vi "Data entry form Post-Assembly.vi"(8 "error in (no error)":errorcluster, 10 "Stack names":T2, 11 "Database Entry in":refnum<class "Database Entry.lvclass">) -> (0 "error out":errorcluster, 2 "Post-Assembly Comments Out":T1, 3 "Database Entry out":refnum<class "Database Entry.lvclass">)   [LabVIEW 2021, in "Database Entry.lvclass"]
uses:
  Database Entry.lvclass
  Components/Stack/Stack.lvclass
panel:
  in  "Submit":bool
  in  "Post-Assembly Comments (If Any)":T3
  # "Note:\nEnsure 320P/320M in stack name to write to their respective tables.\nThis only updates existing \nstacks in postgres."
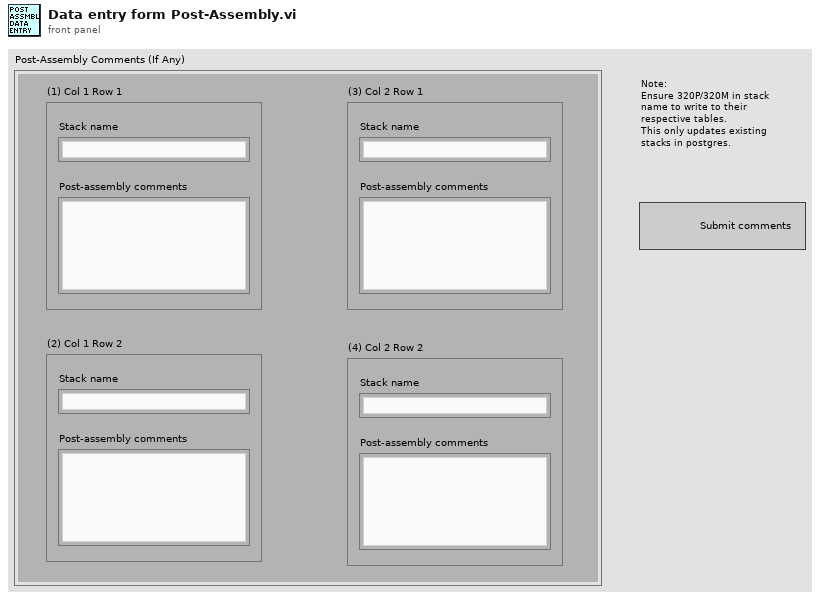
[diagram p1: front panel]
types:
  T1 = cluster{"(1) Tray 1 Pos 1":cluster{"Stack name":string, "Post-assembly comments":string}, "(2) Tray 1 Pos 2":cluster{"Stack name":string, "Post-assembly comments":string}, "(3) Tray 2 Pos 1":cluster{"Stack name":string, "Post-assembly comments":string}, "(4) Tray 2 Pos 2":cluster{"Stack name":string, "Post-assembly comments":string}}
  T2 = cluster{"(1) Tray 1 Pos 1":string, "(2) Tray 1 Pos 2":string, "(3) Tray 2 Pos 1":string, "(4) Tray 2 Pos 2":string}
  T3 = cluster{"(1) Col 1 Row 1":cluster{"Stack name":string, "Post-assembly comments":string}, "(2) Col 1 Row 2":cluster{"Stack name":string, "Post-assembly comments":string}, "(3) Col 2 Row 1":cluster{"Stack name":string, "Post-assembly comments":string}, "(4) Col 2 Row 2":cluster{"Stack name":string, "Post-assembly comments":string}}
  T4 = cluster{"Stack name":string, "Post-assembly comments":string}[]
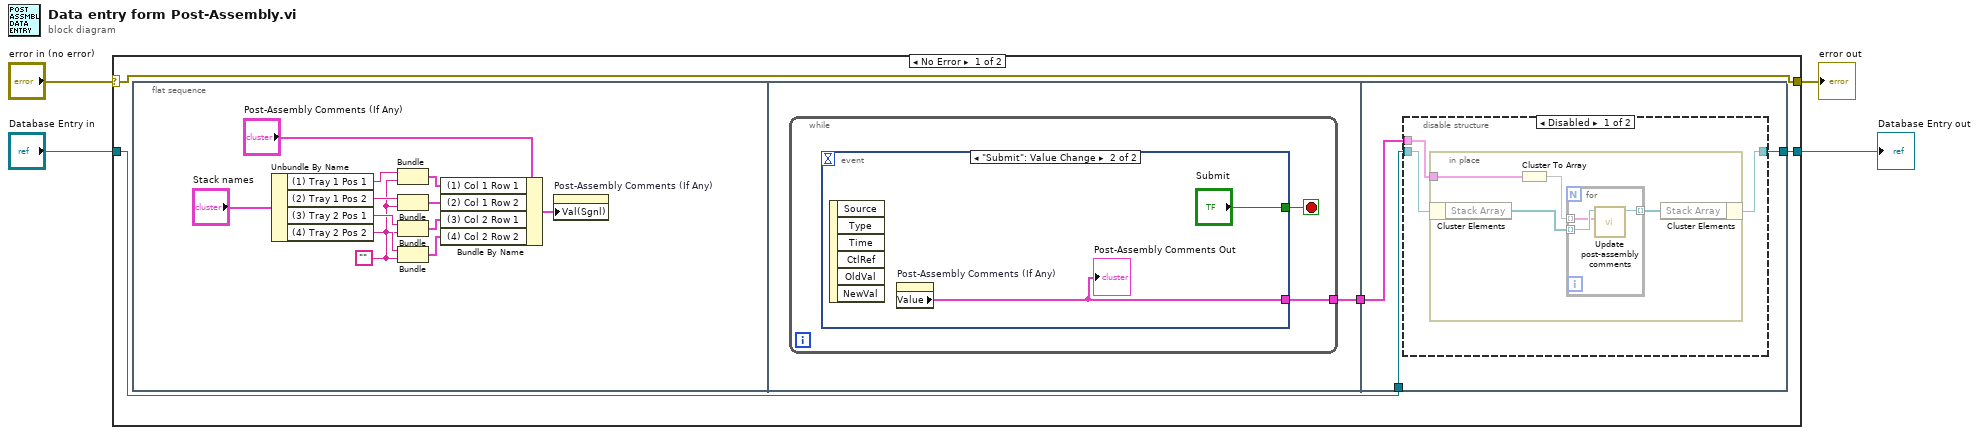
[diagram p0: block diagram]
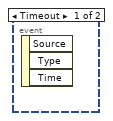
[diagram p2: hidden frame]
diagram:
  n1 = case shown="No Error" "error in (no error)" {
    selector: "error in (no error)" -> [w8 w40]
    tunnel: [w8 w40] -> w3
    tunnel: "Database Entry in" -> [w7 w41]
    tunnel: [w6 w41] -> w1
    frame No Error {
      n2 = flat-sequence {
        tunnel: [w21] -> w5
        tunnel: w7 -> [w28]
        tunnel: [w27] -> w6
        tunnel: w5 -> [w26]
        frame #0 {
          w13 = ""
          n3 = Unbundle By Name("Stack names") -> ("(1) Tray 1 Pos 1"=w19:string, "(2) Tray 1 Pos 2"=w16:string, "(3) Tray 2 Pos 1"=w15:string, "(4) Tray 2 Pos 2"=w14:string)
          n4 = Bundle("(1) Tray 1 Pos 1"=w19, w13) -> (w18:cluster{"(1) Tray 1 Pos 1":string, string})  [unwired: 1 in]
          n5 = Bundle("(2) Tray 1 Pos 2"=w16, w13) -> (w17:cluster{"(2) Tray 1 Pos 2":string, string})  [unwired: 1 in]
          n6 = Bundle("(3) Tray 2 Pos 1"=w15, w13) -> (w12:cluster{"(3) Tray 2 Pos 1":string, string})  [unwired: 1 in]
          n7 = Bundle("(4) Tray 2 Pos 2"=w14, w13) -> (w11:cluster{"(4) Tray 2 Pos 2":string, string})  [unwired: 1 in]
          n8 = Bundle By Name(cluster="Post-Assembly Comments (If Any)", "(1) Col 1 Row 1"=w18, "(2) Col 1 Row 2"=w17, "(3) Col 2 Row 1"=w12, "(4) Col 2 Row 2"=w11) -> (w10:T3)
          n9 = property on="Post-Assembly Comments (If Any)" class="Clust (strict)"("Val(Sgnl)"=w10) -> ()  [unwired: 2 in, 2 out]
        }
        frame #1 {
          n10 = while {
            tunnel: [w22] -> w21
            stop <- w23 stop-if-true
            n11 = event shown="[1] \"Submit\": Value Change" {
              selector: _ -> [_ _]
              dyn-events: _ -> [_ _]
              timeout: _ -> [_ _]
              tunnel: [_ "Submit"] -> w23
              tunnel: [_ w24] -> w22
              event Timeout {
                n12 = event-data() -> ()  [unwired: 1 in, 3 out]
              }
              event "Submit": Value Change {
                n13 = event-data() -> ()  [unwired: 1 in, 6 out]
                n14 = property on="Post-Assembly Comments (If Any)" class="Clust (strict)"() -> ("Value"=w24:T1)  [unwired: 2 in, 2 out]
                "Post-Assembly Comments Out" <- w24
              }
            }
          }
        }
        frame #2 {
          n15 = disable-structure shown="Disabled" {
            disable-tunnel: w28 -> [w31 w39]
            disable-tunnel: [w30 w39] -> w27
            disable-tunnel: w26 -> [w29 _]
            frame Disabled {
              n16 = in-place {
                in-place-border: w29 -> [w33]
                n17 = in-place-cluster #1(w31) -> ("Stack Array"=w35:refnum<class "Stack.lvclass">[])
                n18 = Cluster To Array(cluster=w33) -> (array=w32:T4)
                n19 = for {
                  tunnel: w35 -> [w38] mode=indexing
                  tunnel: [w37] -> w34 mode=indexing
                  tunnel: w32 -> [w36] mode=indexing
                  n20 = call "Update post-assembly comments.vi"("Tray N Pos M"=w36, "Stack in"=w38) -> ("Stack out"=w37:refnum<class "Stack.lvclass">)  [unwired: 8 in, 1 out]
                }
                n21 = in-place-cluster #1("Stack Array"=w34) -> (w30:refnum<class "Database Entry.lvclass">)
              }
            }
            frame Enabled {
            }
          }
        }
      }
    }
    frame Error {
    }
  }
  "Database Entry out" <- w1
  "error out" <- w3
